vi "Check Corruption Queue.vi"(11 "input string":string) -> (1 "Remaining string":string[](array[string]), 2 "Corrupted?":bool, 3 "Score":i32, 5 "Invalid Character":bool)   [LabVIEW 2019, in "Day 10.lvlib"]
uses:
  Day 10.lvlib
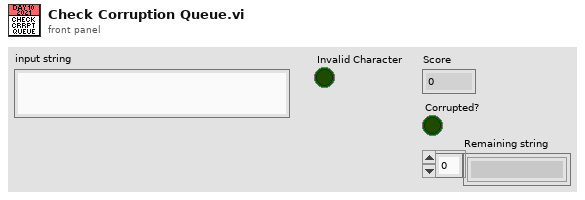
[diagram p1: front panel]
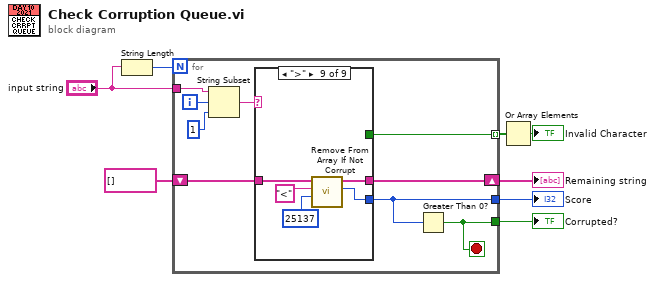
[diagram p0: block diagram]
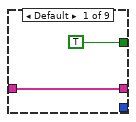
[diagram p2: hidden frame]
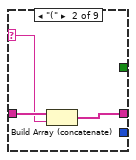
[diagram p3: hidden frame]
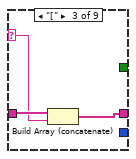
[diagram p4: hidden frame]
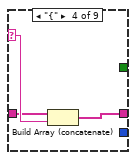
[diagram p5: hidden frame]
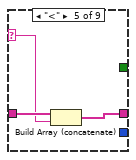
[diagram p6: hidden frame]
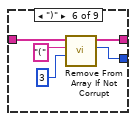
[diagram p7: hidden frame]
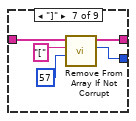
[diagram p8: hidden frame]
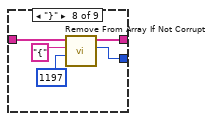
[diagram p9: hidden frame]
diagram:
  n1 = String Length(string="input string") -> (length=w8:i32)
  n2 = for {
    N: w8 -> [_]
    tunnel: "input string" -> [w17]
    shift-right: [w12] -> w1
    shift-left: string[] [] -> [w13]
    tunnel: [w11] -> w5 mode=indexing
    tunnel: [w10] -> w2
    tunnel: [w9] -> w3
    i -> [w16]
    stop <- w9 stop-if-true
    n3 = String Subset(string=w17, offset (0)=w16, length (rest)=1 ("length (rest)")) -> (substring=w14:string)
    n4 = case shown="\">\"" w14 {
      selector: w14 -> [_ w21 w24 w28 w30 _ _ _ _]
      tunnel: w13 -> [w19 w22 w25 w27 w31 w35 w40 w45 w50]
      tunnel: [w19 w20 w23 w26 w29 w34 w39 w44 w49] -> w12
      tunnel: [TRUE _ _ _ _ _ _ _ _] -> w11
      tunnel: [_ _ _ _ _ w33 w38 w43 w48] -> w10
      frame Default {
      }
      frame "(" {
        n5 = Build Array (concatenate)(w22, w21) -> (w20:string[])
      }
      frame "[" {
        n6 = Build Array (concatenate)(w25, w24) -> (w23:string[])
      }
      frame "{" {
        n7 = Build Array (concatenate)(w27, w28) -> (w26:string[])
      }
      frame "<" {
        n8 = Build Array (concatenate)(w31, w30) -> (w29:string[])
      }
      frame ")" {
        n9 = call "Remove From Array If Not Corrupt.vi"("Score"=3, "Expected Char"="(" ("y"), "Array in"=w35) -> ("Score"=w33:i32, "Array out"=w34:string[])  [unwired: 7 in]
      }
      frame "]" {
        n10 = call "Remove From Array If Not Corrupt.vi"("Score"=57, "Expected Char"="[" ("y"), "Array in"=w40) -> ("Score"=w38:i32, "Array out"=w39:string[])  [unwired: 7 in]
      }
      frame "}" {
        n11 = call "Remove From Array If Not Corrupt.vi"("Score"=1197, "Expected Char"="{" ("y"), "Array in"=w45) -> ("Score"=w43:i32, "Array out"=w44:string[])  [unwired: 7 in]
      }
      frame ">" {
        n12 = call "Remove From Array If Not Corrupt.vi"("Score"=25137, "Expected Char"="<" ("y"), "Array in"=w50) -> ("Score"=w48:i32, "Array out"=w49:string[])  [unwired: 7 in]
      }
    }
    n13 = Greater Than 0?(x=w10) -> (x > 0?=w9:bool)
  }
  "Corrupted?" <- w3
  "Score" <- w2
  "Remaining string" <- w1
  n14 = Or Array Elements(Boolean array=w5) -> (logical OR=→"Invalid Character":bool)
